vi "LinkedGUI.vi"() -> ()   [LabVIEW 2020, in "VolatusScratch.lvlib"]
uses:
  VolatusScratch.lvlib
panel:
  out "Ox_Level_3":cluster{"Color":u32, "Value":dbl}
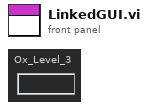
[diagram p1: front panel]
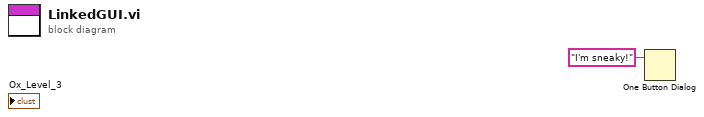
[diagram p0: block diagram]
diagram:
  n1 = One Button Dialog(message="I'm sneaky!") -> ()  [unwired: 1 in, 1 out]
